vi "EnteringState.vi"(0 "StateIn":T6 {"ILoad" format="%_6g"; "Fault Registers" format="%016x"; "VLoad" format="%_6g"; "VDCLink" format="%_6g"; "Detected Frequency" format="%1_6g"}, 1 "Interfaces":T1, 11 "error in (no error)":errorcluster) -> (4 "StateOut":T6 {"ILoad" format="%_6g"; "Fault Registers" format="%016x"; "VLoad" format="%_6g"; "VDCLink" format="%_6g"; "Detected Frequency" format="%1_6g"}, 15 "error out":errorcluster)   [LabVIEW 2017, in "AppStateMachine runtime.lvclass"]
uses:
  AppStateMachine runtime.lvclass
  State.ctl
  StateId.ctl
  LED_Color.ctl
  Interfaces.ctl
  <vilib>/NI/NI JSONRPC Server Framework/Classes/Server/JSONRPC Server.lvclass
  <instrlib>/_niInstr/Instruction Framework/v1/Host/Instruction Target/niInstr Instruction Target v1 Host.lvclass
  <instrlib>/_niInstr/Instruction Framework/v1/Host/Instruction Framework Context/niInstr Instruction Framework Context v1 Host.lvclass
  FPGA/FPGAtypedef.ctl
  <vilib>/NI/PowerElectronicsControl/ThreePhasePLL/Interface/InterfaceRef.ctl
  <vilib>/NI/PowerElectronicsControl/ActiveFrontEnd/AFE_Interface/InterfaceRef.ctl
  <vilib>/NI/PowerElectronicsControl/Buck-Boost/RealTime/Interface.ctl
  <vilib>/NI/PowerElectronicsControl/ActiveFrontEnd/AFE_Interface/Setpoints.ctl
  <vilib>/Utility/error.llb/Error Cluster From Error Code.vi
  <vilib>/rvi/errors/niLvFpgaAdjustHostInterfaceError.vi
  <vilib>/rvi/interface/nirviReadWriteControl/nirviReadWriteControl.xnode
  NiFpgaLv.dll
  <vilib>/rvi/interface/Simulation/niFpgaSimulationCallBeginRW.vi
  <vilib>/NI/PowerElectronicsControl/Buck-Boost/RealTime/BuckBoostInterface.lvlib
  <vilib>/NI/PowerElectronicsControl/ActiveFrontEnd/AFE_Interface/AFE_interface.lvlib
  <vilib>/NI/PowerElectronicsControl/ThreePhasePLL/Interface/ThreePhasePLLInterface.lvlib
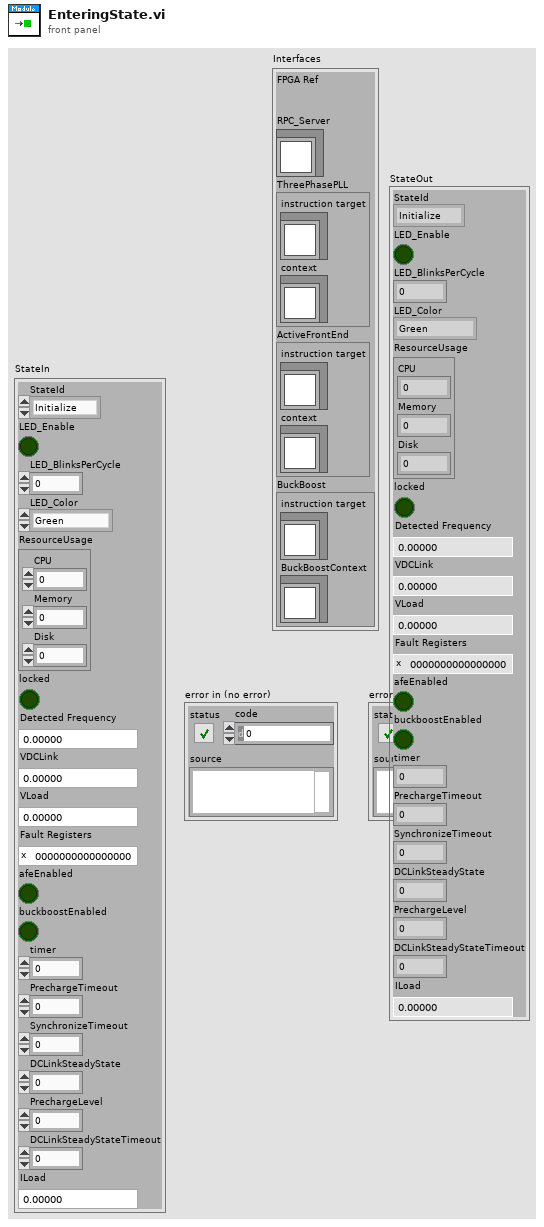
[diagram p1: front panel]
types:
  T1 = typedef "AppStateMachine runtime.lvclass/Interfaces.ctl" = cluster{"FPGA Ref":T2, "RPC_Server":refnum<class "JSONRPC Server.lvclass">, "ThreePhasePLL":T3, "ActiveFrontEnd":T4, "BuckBoost":T5}
  T2 = typedef "AppStateMachine runtime.lvclass/FPGAtypedef.ctl" = refnum<k20>
  T3 = typedef "ThreePhasePLLInterface.lvlib/InterfaceRef.ctl" = cluster{"instruction target":refnum<class "niInstr Instruction Target v1 Host.lvclass">, "context":refnum<class "niInstr Instruction Framework Context v1 Host.lvclass">}
  T4 = typedef "AFE_interface.lvlib/InterfaceRef.ctl" = cluster{"instruction target":refnum<class "niInstr Instruction Target v1 Host.lvclass">, "context":refnum<class "niInstr Instruction Framework Context v1 Host.lvclass">}
  T5 = typedef "BuckBoostInterface.lvlib/Interface.ctl" = cluster{"instruction target":refnum<class "niInstr Instruction Target v1 Host.lvclass">, "BuckBoostContext":refnum<class "niInstr Instruction Framework Context v1 Host.lvclass">}
  T6 = typedef "AppStateMachine runtime.lvclass/State.ctl" = cluster{"StateId":T7, "LED_Enable":bool, "LED_BlinksPerCycle":i32, "LED_Color":T8, "ResourceUsage":cluster{"CPU":dbl, "Memory":dbl, "Disk":dbl}, "locked":bool, "Detected Frequency":dbl, "VDCLink":dbl, "VLoad":dbl, "Fault Registers":u64, "afeEnabled":bool, "buckboostEnabled":bool, "timer":u32, "PrechargeTimeout":u32, "SynchronizeTimeout":u32, "DCLinkSteadyState":dbl, "PrechargeLevel":dbl, "DCLinkSteadyStateTimeout":u32, "ILoad":dbl}
  T7 = typedef "AppStateMachine runtime.lvclass/StateId.ctl" = enum16{"Initialize", "Idle", "TunePLL", "TuneAFE", "TuneBuckBoost", "Precharge", "Synchronize", "Ready", "EnableAFE", "EnableBuckBoost", "Powered", "SafeState", "UnrecoverableSafeState"}
  T8 = typedef "AppStateMachine runtime.lvclass/LED_Color.ctl" = enum16{"Green", "Yellow"}
  T9 = typedef "AFE_interface.lvlib/Setpoints.ctl" = enum16{"VDCLink", "Q", "Powerfactor"}
  T10 = typedef "AFE_interface.lvlib/Feedback.ctl" = cluster{"VDClink":dbl, "P":dbl, "Q":dbl, "pf":dbl}
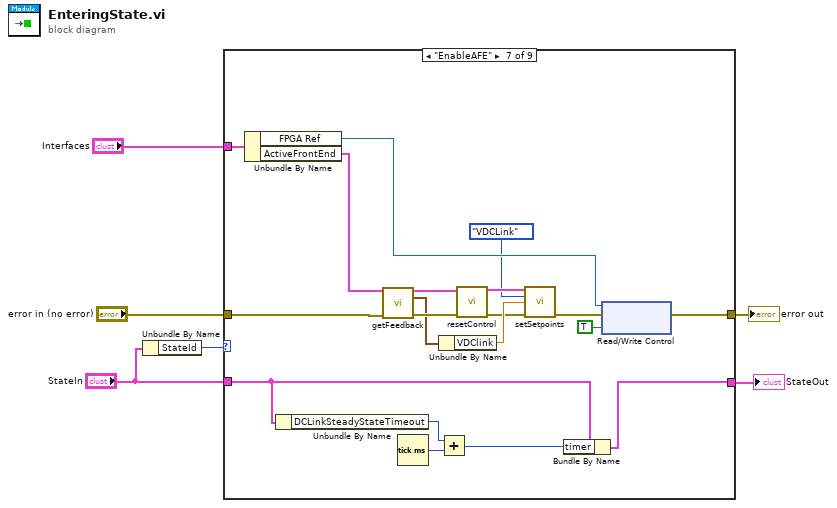
[diagram p0: block diagram]
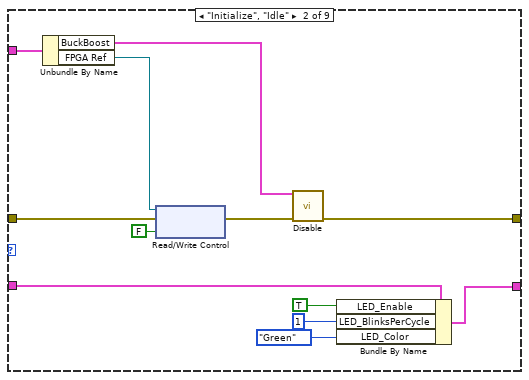
[diagram p3: hidden frame]
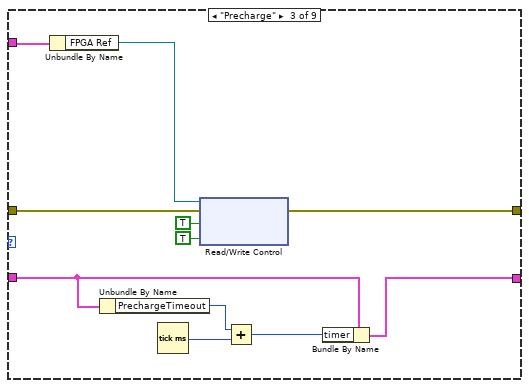
[diagram p4: hidden frame]
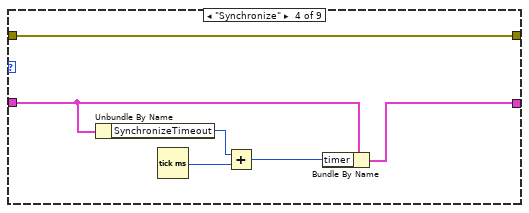
[diagram p5: hidden frame]
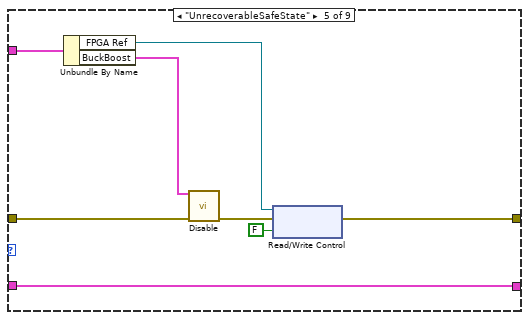
[diagram p6: hidden frame]
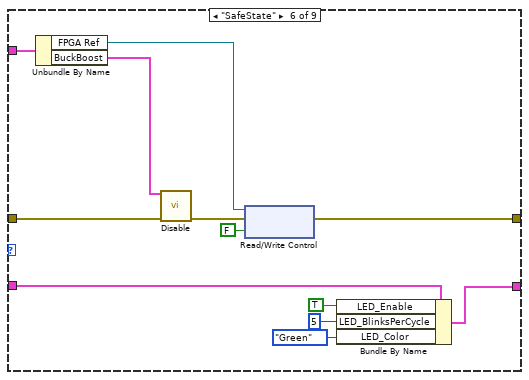
[diagram p7: hidden frame]
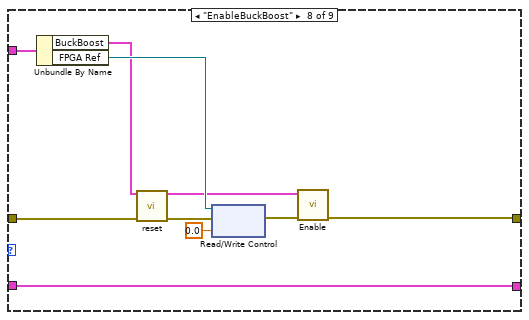
[diagram p8: hidden frame]
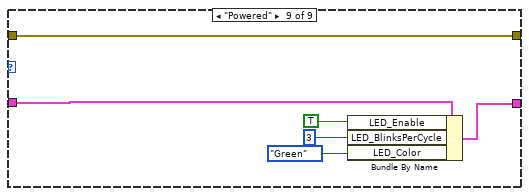
[diagram p9: hidden frame]
diagram:
  n1 = Unbundle By Name("StateIn") -> ("StateId"=w4:T7)
  n2 = case shown="\"EnableAFE\"" w4 {
    tunnel: "error in (no error)" -> [w8 w14 w30 w32 w39 w48 w71 w84 w88]
    tunnel: [w8 w9 w29 w32 w38 w46 w75 w78 w88] -> w6
    tunnel: "StateIn" -> [w7 w20 w22 w34 w45 w57 w59 w77 w87]
    tunnel: [w7 w16 w21 w33 w45 w53 w58 w77 w89] -> w2
    tunnel: "Interfaces" -> [_ w15 w31 _ w40 w51 w76 w86 _]
    frame Default {
    }
    frame "Initialize", "Idle" {
      n3 = Unbundle By Name(w15) -> ("BuckBoost"=w10:T5, "FPGA Ref"=w13:T2)
      n4 = xnode "Read/Write Control"("FPGA VI Reference In"=w13, "error in"=w14, "enableAFE"=FALSE) -> ("error out"=w11:errorcluster)  [unwired: 1 out]
      n5 = call <vilib>:"Disable.vi"("Interface in"=w10, "error in (no error)"=w11) -> ("error out"=w9:errorcluster)  [unwired: 12 in, 1 out]
      n6 = Bundle By Name(cluster=w20, "LED_Enable"=TRUE, "LED_BlinksPerCycle"=1, "LED_Color"=LED_Color."Green") -> (w16:T6)
    }
    frame "Precharge" {
      n7 = Unbundle By Name(w31) -> ("FPGA Ref"=w28:T2)
      n8 = Unbundle By Name(w22) -> ("PrechargeTimeout"=w24:u32)
      n9 = Tick Count (ms)() -> (millisecond timer value=w25:u32)
      n10 = xnode "Read/Write Control"("FPGA VI Reference In"=w28, "error in"=w30, "PrechargeAFE"=TRUE, "MainContactor"=TRUE) -> ("error out"=w29:errorcluster)  [unwired: 1 out]
      n11 = Add(x=w24, y=w25) -> (x+y=w23:u32)
      n12 = Bundle By Name(cluster=w22, "timer"=w23) -> (w21:T6)
    }
    frame "Synchronize" {
      n13 = Unbundle By Name(w34) -> ("SynchronizeTimeout"=w36:u32)
      n14 = Tick Count (ms)() -> (millisecond timer value=w37:u32)
      n15 = Add(x=w36, y=w37) -> (x+y=w35:u32)
      n16 = Bundle By Name(cluster=w34, "timer"=w35) -> (w33:T6)
    }
    frame "UnrecoverableSafeState" {
      n17 = Unbundle By Name(w40) -> ("FPGA Ref"=w43:T2, "BuckBoost"=w41:T5)
      n18 = call <vilib>:"Disable.vi"("Interface in"=w41, "error in (no error)"=w39) -> ("error out"=w42:errorcluster)  [unwired: 12 in, 1 out]
      n19 = xnode "Read/Write Control"("FPGA VI Reference In"=w43, "error in"=w42, "enableAFE"=FALSE) -> ("error out"=w38:errorcluster)  [unwired: 1 out]
    }
    frame "SafeState" {
      n20 = Unbundle By Name(w51) -> ("FPGA Ref"=w50:T2, "BuckBoost"=w47:T5)
      n21 = call <vilib>:"Disable.vi"("Interface in"=w47, "error in (no error)"=w48) -> ("error out"=w49:errorcluster)  [unwired: 12 in, 1 out]
      n22 = xnode "Read/Write Control"("FPGA VI Reference In"=w50, "error in"=w49, "enableAFE"=FALSE) -> ("error out"=w46:errorcluster)  [unwired: 1 out]
      n23 = Bundle By Name(cluster=w57, "LED_Enable"=TRUE, "LED_BlinksPerCycle"=5, "LED_Color"=LED_Color."Green") -> (w53:T6)
    }
    frame "EnableAFE" {
      n24 = Unbundle By Name(w76) -> ("FPGA Ref"=w74:T2, "ActiveFrontEnd"=w69:T4)
      n25 = Unbundle By Name(w59) -> ("DCLinkSteadyStateTimeout"=w61:u32)
      n26 = call <vilib>:"getFeedback.vi"("Interface in"=w69, "error in"=w71) -> ("Interface out"=w68:T4, "feedback"=w67:T10, "error out"=w70:errorcluster)  [unwired: 11 in]
      n27 = Tick Count (ms)() -> (millisecond timer value=w62:u32)
      n28 = Unbundle By Name(w67) -> ("VDClink"=w65:dbl)
      n29 = Add(x=w61, y=w62) -> (x+y=w60:u32)
      n30 = call <vilib>:"resetControl.vi"("Interface in"=w68, "error in"=w70) -> ("Interface out"=w72:T4, "error out"=w64:errorcluster)  [unwired: 12 in]
      n31 = call <vilib>:"setSetpoints.vi"("Interface in"=w72, "Setpoint"=Setpoints."VDCLink", "Value"=w65, "error in"=w64) -> ("error out"=w63:errorcluster)  [unwired: 10 in, 1 out]
      n32 = Bundle By Name(cluster=w59, "timer"=w60) -> (w58:T6)
      n33 = xnode "Read/Write Control"("FPGA VI Reference In"=w74, "error in"=w63, "enableAFE"=TRUE) -> ("error out"=w75:errorcluster)  [unwired: 1 out]
    }
    frame "EnableBuckBoost" {
      n34 = Unbundle By Name(w86) -> ("BuckBoost"=w83:T5, "FPGA Ref"=w85:T2)
      n35 = call <vilib>:"reset.vi"("Interface in"=w83, "error in (no error)"=w84) -> ("Interface out"=w79:T5, "error out"=w82:errorcluster)  [unwired: 12 in]
      n36 = xnode "Read/Write Control"("FPGA VI Reference In"=w85, "error in"=w82, "I_setpt"=sgl 0.0) -> ("error out"=w80:errorcluster)  [unwired: 1 out]
      n37 = call <vilib>:"Enable.vi"("Interface in"=w79, "error in (no error)"=w80) -> ("error out"=w78:errorcluster)  [unwired: 12 in, 1 out]
    }
    frame "Powered" {
      n38 = Bundle By Name(cluster=w87, "LED_Enable"=TRUE, "LED_BlinksPerCycle"=3, "LED_Color"=LED_Color."Green") -> (w89:T6)
    }
  }
  "error out" <- w6
  "StateOut" <- w2
